vi "Write All Variables.vi"(8 "error in (no error)":errorcluster, 10 "Analys. vars.":T1, 11 "Analysis params in":refnum<class "CV-Analysis.lvclass">) -> (0 "error out":errorcluster, 3 "Analysis params out":refnum<class "CV-Analysis.lvclass">)   [LabVIEW 2013, in "CameraVision.lvlib" / "CV-Analysis.lvclass"]
uses:
  CV-Analysis.lvclass
  Analysis-variables.ctl
  Characteristics-cluster.ctl
  CV-Analysis.lvclass/CV-Analysis.ctl
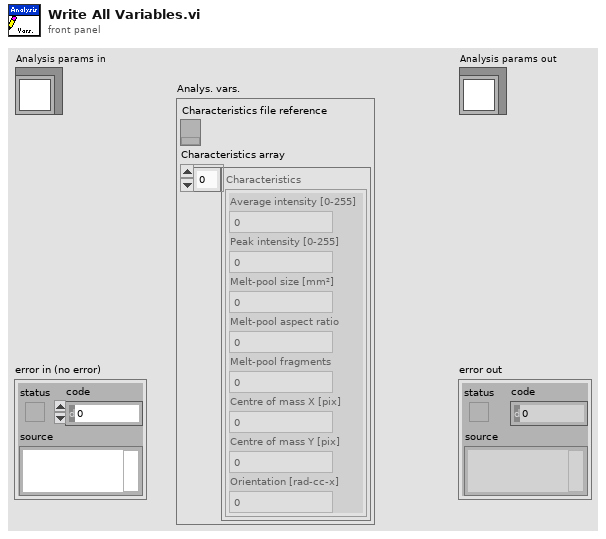
[diagram p1: front panel]
types:
  T1 = typedef "CameraVision.lvlib/CV-Analysis.lvclass/Analysis-variables.ctl" = cluster{"Characteristics file reference":refnum<k34>, "Characteristics array":T2[]}
  T2 = typedef "CameraVision.lvlib/CV-Analysis.lvclass/Characteristics-cluster.ctl" = cluster{"Average intensity":dbl, "Peak intensity":dbl, "Melt-pool size":dbl, "Melt-pool aspect ratio":dbl, "Melt-pool fragments":dbl, "Centre of mass X":dbl, "Centre of mass Y":dbl, "Orientation":dbl}
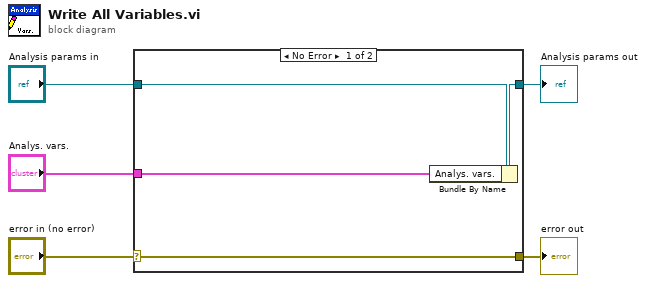
[diagram p0: block diagram]
diagram:
  n1 = case shown="No Error" "error in (no error)" {
    selector: "error in (no error)" -> [w9 w10]
    tunnel: [w9 w10] -> w4
    tunnel: [w7 w11] -> w2
    tunnel: "Analysis params in" -> [w8 w11]
    tunnel: "Analys. vars." -> [w6 _]
    frame No Error {
      n2 = Bundle By Name(cluster=w8, "Analys. vars."=w6) -> (w7:refnum<class "CV-Analysis.lvclass">)
    }
    frame Error {
    }
  }
  "error out" <- w4
  "Analysis params out" <- w2
